vi "Read String.vi"(8 "error in (no error)":errorcluster, 11 "string in":refnum<class "string.lvclass">) -> (0 "error out":errorcluster, 2 "Value":string, 3 "string out":refnum<class "string.lvclass">)   [LabVIEW 2020, in "Protobuf RAW.lvlib" / "string.lvclass"]
uses:
  string.lvclass
  string.lvclass/string.ctl
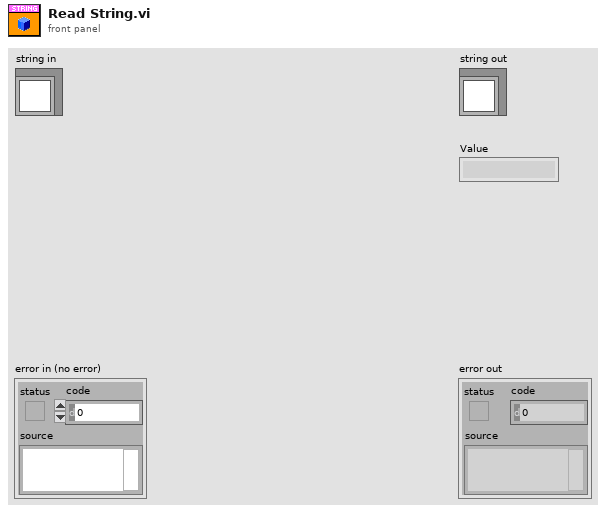
[diagram p1: front panel]
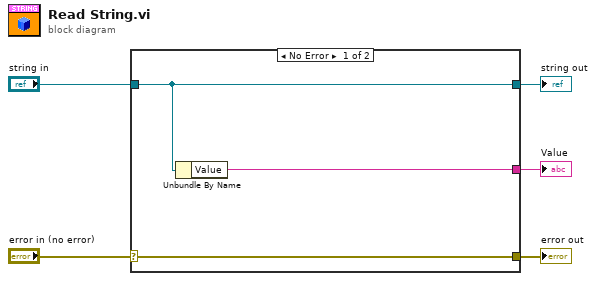
[diagram p0: block diagram]
diagram:
  n1 = case shown="No Error" "error in (no error)" {
    selector: "error in (no error)" -> [w8 w9]
    tunnel: [w8 w9] -> w4
    tunnel: [w7 w10] -> w2
    tunnel: "string in" -> [w7 w10]
    tunnel: [w6 _] -> w1
    frame No Error {
      n2 = Unbundle By Name(w7) -> ("Value"=w6:string)
    }
    frame Error {
    }
  }
  "error out" <- w4
  "string out" <- w2
  "Value" <- w1
